vi "Add Page.vi"(4 "Replace If Exists? (T)":bool=TRUE, 5 "Template (\"\")":string, 6 "Paths":string[](array[string]), 7 "VI Refnum (NaN)":refnum<vi>, 8 "error in (no error)":errorcluster, 9 "Content-Type":string, 10 "Content":string, 11 "Endpoint":string) -> (0 "error out":errorcluster)   [LabVIEW 2021, in "HttpServer.lvlib"]
uses:
  HttpServer.lvlib
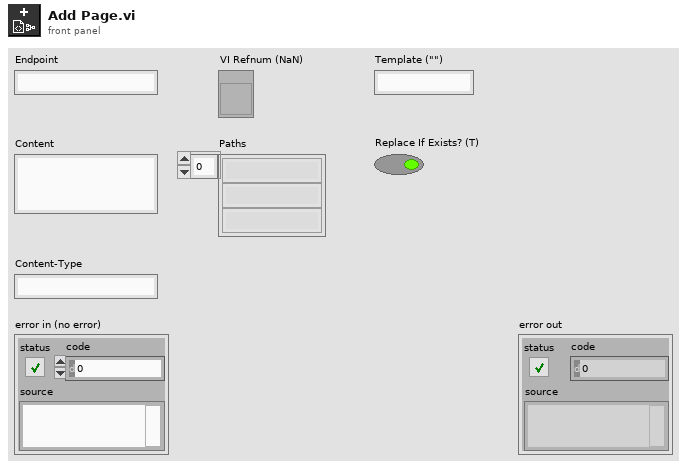
[diagram p1: front panel]
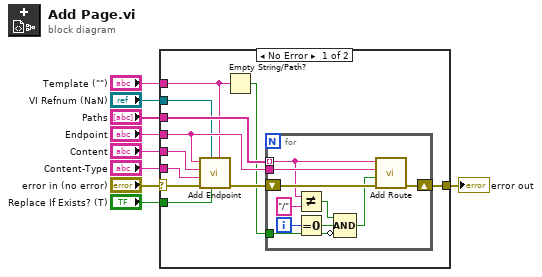
[diagram p0: block diagram]
diagram:
  n1 = case shown="No Error" "error in (no error)" {
    selector: "error in (no error)" -> [w20 w31]
    tunnel: [w18 w31] -> w8
    tunnel: "Content" -> [w17 _]
    tunnel: "Content-Type" -> [w16 _]
    tunnel: "VI Refnum (NaN)" -> [w12 _]
    tunnel: "Endpoint" -> [w15 _]
    tunnel: "Paths" -> [w14 _]
    tunnel: "Replace If Exists? (T)" -> [w13 _]
    tunnel: "Template (\"\")" -> [w11 _]
    frame No Error {
      n2 = call "Add Endpoint.vi"("Template (\"\"=Static File)"=w11, "Replace if exists? (T)"=w13, "VI Refnum in"=w12, "error in (no error)"=w20, "Content-Type"=w16, "Content"=w17, "Endpoint"=w15) -> ("error out"=w19:errorcluster)  [unwired: 3 in, 1 out]
      n3 = Empty String/Path?(string/path=w11) -> (empty?=w10:bool)
      n4 = for {
        tunnel: w15 -> [w28]
        shift-right: [w29] -> w18
        shift-left: w19 -> [w30]
        tunnel: w14 -> [w24] mode=indexing
        tunnel: w10 -> [w21]
        i -> [w27]
        n5 = Not Equal?(x=w24, y="/") -> (x != y?=w22:bool)
        n6 = Equal To 0?(x=w27) -> (x = 0?=w26:bool)
        n7 = Compound Arithmetic op=AND(w22, w26, invert w21) -> (w25:bool)
        n8 = call "Add Route.vi"("error in (no error)"=w30, "Navbar Page? (F)"=w25, "Endpoint"=w28, "Path"=w24) -> ("error out"=w29:errorcluster)  [unwired: 7 in]
      }
    }
    frame Error {
    }
  }
  "error out" <- w8
